vi "scan_2d_retrace_axis.vi"(8 "error in (no error)":errorcluster, 9 "Retrace Time (s)":dbl, 10 "axis":T1, 11 "scan_2d in":refnum<class "scan_2d.lvclass">) -> (0 "error out":errorcluster, 3 "scan_2d out":refnum<class "scan_2d.lvclass">)   [LabVIEW 2015, in "scan_2d.lvclass"]
uses:
  scan_2d.lvclass
  scan2d_axistypes_tdef.ctl
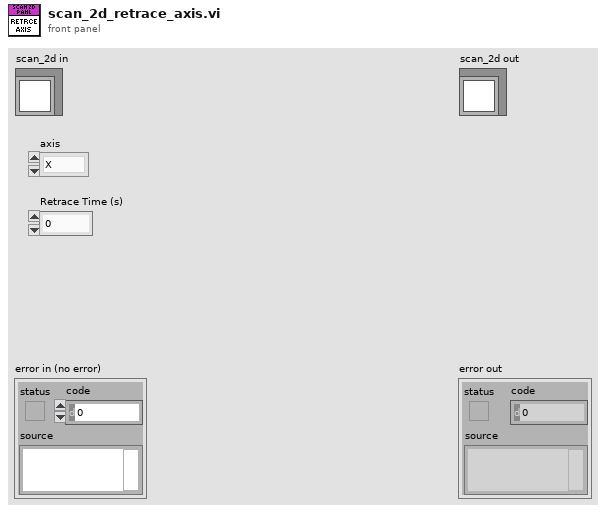
[diagram p1: front panel]
types:
  T1 = typedef "scan2d_axistypes_tdef.ctl" = enum16{"X", "Y"}
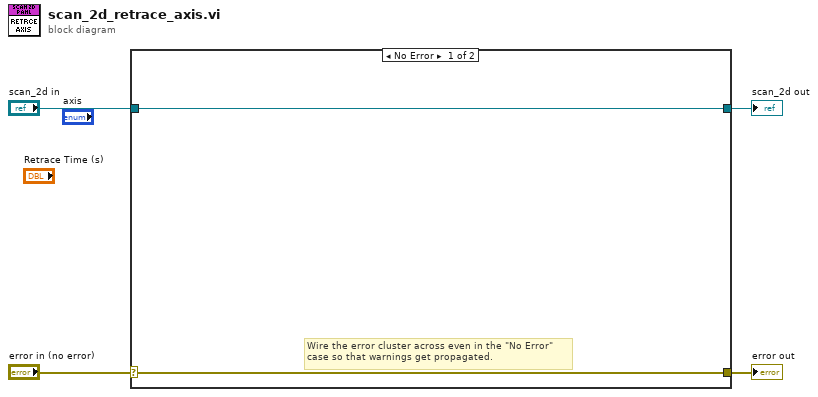
[diagram p0: block diagram]
diagram:
  n1 = case shown="No Error" "error in (no error)" {
    selector: "error in (no error)" -> [w5 w8]
    tunnel: [w5 w8] -> w3
    tunnel: [w6 w7] -> w1
    tunnel: "scan_2d in" -> [w6 w7]
    frame No Error {
      # "Wire the error cluster across even in the \"No Error\"\ncase so that warnings get propagated."
    }
    frame Error {
    }
  }
  "error out" <- w3
  "scan_2d out" <- w1
